vi "tform_t2c.vi"(0 "X_TIRF":sgl, 1 "Y_TIRF":sgl, 2 "X_Stage":dbl, 3 "Y_Stage":dbl, 8 "Nb pts X&Y":u32) -> (9 "Pixel index in cfc":dbl[](array[numeric]), 12 "Scanning parameters":T1, 13 "Y_cfc":dbl, 17 "X_cfc":dbl)   [LabVIEW 2015]
uses:
  <vilib>/Analysis/Matrix/Datatypes/RealMatrix.ctl
  <vilib>/Analysis/baseanly.llb/Vector x A.vi
  <vilib>/Analysis/Matrix/NI_Matrix.lvlib
  <vilib>/Analysis/NI_AALBase.lvlib
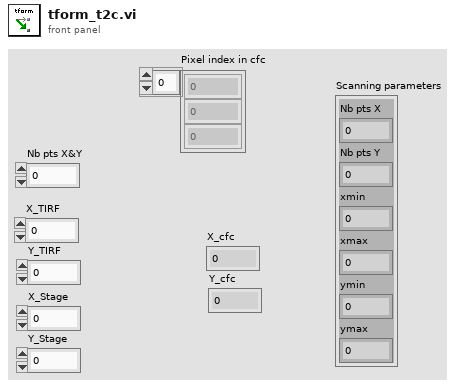
[diagram p1: front panel]
types:
  T1 = cluster{"Nb pts X":u32, "Nb pts Y":u32, "xmin":dbl, "xmax":dbl, "ymin":dbl, "ymax":dbl}
  T2 = typedef "NI_Matrix.lvlib/RealMatrix.ctl" = dbl[][]
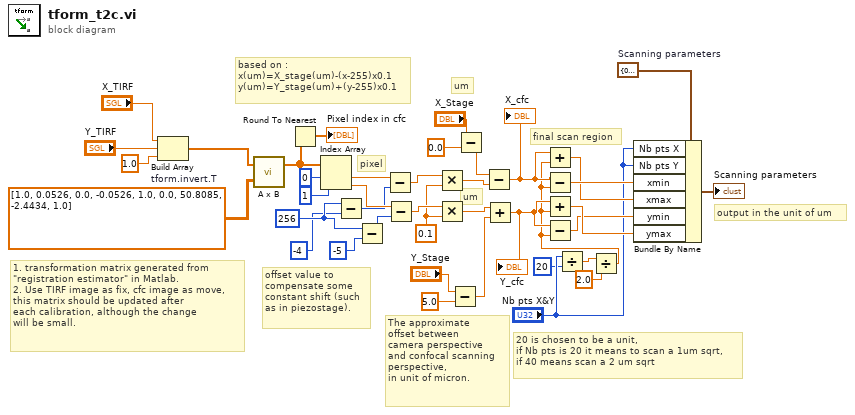
[diagram p0: block diagram]
diagram:
  w3 = 256
  w19 = T1 {"Nb pts X"=0, "Nb pts Y"=0, "xmin"=0.0, "xmax"=0.0, "ymin"=0.0, "ymax"=0.0}  # Scanning parameters
  w21 = 0.1
  w39 = T2 [[1.0, 0.0526, 0.0], [-0.0526, 1.0, 0.0], [50.8085, -2.4434, 1.0]]  # tform.invert.T
  # "The approximate \noffset between \ncamera perspective \nand confocal scanning\nperspective, \nin unit of micron."
  # "offset value to \ncompensate some \nconstant shift (such\nas in piezostage)."
  # "output in the unit of um"
  # "pixel"
  # "um"
  # "um"
  # "20 is chosen to be a unit, \nif Nb pts is 20 it means to scan a 1um sqrt, \nif 40 means scan a 2 um sqrt"
  # "1. transformation matrix generated from \n\"registration estimator\" in Matlab.\n2. Use TIRF image as fix, cfc image as move,\nthis matrix should be updated after \neach calibration, although the change \nwill be small."
  # "final scan region"
  # "based on :\nx(um)=X_stage(um)-(x-255)x0.1\ny(um)=Y_stage(um)+(y-255)x0.1"
  n1 = Build Array("X_TIRF", "Y_TIRF", sgl 1.0 ("element")) -> (w38:sgl[])
  n2 = call-poly <vilib>:"A x B.vi"("Matrix A"=w39, "Vector V'"=w38) -> ("V' x A"=w35:dbl[])  [unwired: 1 out]
  n3 = Round To Nearest(number=w35) -> (nearest integer value=→"Pixel index in cfc":dbl[])
  n4 = Index Array(array=w35, index #1=0 ("index"), index #2=1 ("index")) -> (element #1=w31:dbl, element #2=w32:dbl)
  n5 = Subtract(x=w3, y=-4 ("X_offset")) -> (x-y=w5:i32)
  n6 = Subtract(x=w3, y=-5 ("Y_offset")) -> (x-y=w4:i32)
  n7 = Subtract(x=w31, y=w5) -> (x-y=w30:dbl)
  n8 = Subtract(x=w32, y=w4) -> (x-y=w29:dbl)
  n9 = Multiply(x=w30, y=w21) -> (x*y=w28:dbl)
  n10 = Multiply(x=w29, y=w21) -> (x*y=w27:dbl)
  n11 = Subtract(x="Y_Stage", y=5.0) -> (x-y=w24:dbl)
  n12 = Subtract(x="X_Stage", y=0.0) -> (x-y=w7:dbl)
  n13 = Subtract(x=w7, y=w28) -> (x-y=w23:dbl)
  "X_cfc" <- w23
  n14 = Add(x=w27, y=w24) -> (x+y=w22:dbl)
  "Y_cfc" <- w22
  n15 = Divide(x="Nb pts X&Y", y=u32 20) -> (x/y=w9:dbl)
  n16 = Divide(x=w9, y=2.0) -> (x/y=w10:dbl)
  n17 = Add(x=w23, y=w10) -> (x+y=w18:dbl)
  n18 = Subtract(x=w23, y=w10) -> (x-y=w20:dbl)
  n19 = Add(x=w22, y=w10) -> (x+y=w17:dbl)
  n20 = Subtract(x=w22, y=w10) -> (x-y=w14:dbl)
  n21 = Bundle By Name(cluster=w19, "Nb pts X"="Nb pts X&Y", "Nb pts Y"="Nb pts X&Y", "xmin"=w20, "xmax"=w18, "ymin"=w14, "ymax"=w17) -> (→"Scanning parameters":T1)
